vi "HTMLtoImage.vi"(8 "error in (no error)":errorcluster, 11 "body":string) -> (3 "new picture":picture)   [LabVIEW 2019]
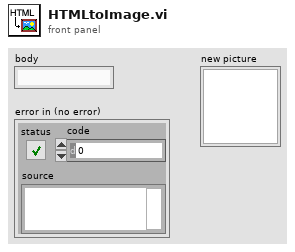
[diagram p1: front panel]
types:
  T1 = typedef "imagedata.ctl" = cluster{"image type":i32, "image depth":i32, "image":u8[], "mask":u8[], "colors":u32[], "Rectangle":cluster{"left":i16, "top":i16, "right":i16, "bottom":i16}}
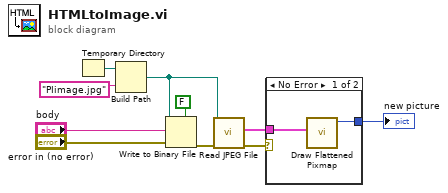
[diagram p0: block diagram]
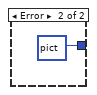
[diagram p2: hidden frame]
diagram:
  n1 = Temporary Directory() -> (w9:path)
  n2 = Build Path(base path=w9, name or relative path="PIimage.jpg") -> (appended path=w7:path)
  n3 = Write to Binary File(file (use dialog)=w7, data="body", error in="error in (no error)", 5:FALSE ("prepend array or string size? (T)")) -> (error out=w1:errorcluster)  [unwired: 2 in, 2 out]
  n4 = call <vilib>:"Read JPEG File.vi"("error in (no error)"=w1, "path to JPEG file"=w7) -> ("error out"=w4:errorcluster, "image data"=w2:T1)  [unwired: 7 in, 1 out]
  n5 = case shown="No Error" w4 {
    tunnel: w2 -> [w12 _]
    tunnel: [w11 picture data[5B] ("new picture")] -> w3
    frame No Error {
      n6 = call <vilib>:"Draw Flattened Pixmap.vi"("image data"=w12) -> ("new picture"=w11:picture)  [unwired: 8 in]
    }
    frame Error {
    }
  }
  "new picture" <- w3
